vi "Get Track Info.vi"(8 "error in (no error)":errorcluster, 10 "Track Index":i32, 11 "midi file in":refnum<class "midi file.lvclass">) -> (0 "error out":errorcluster, 1 "Track Name":string, 2 "Track Info":T1, 3 "midi file out":refnum<class "midi file.lvclass">)   [LabVIEW 2020, in "midi file.lvclass"]
uses:
  midi file.lvclass
  track info.ctl
  midi file.lvclass/midi file.ctl
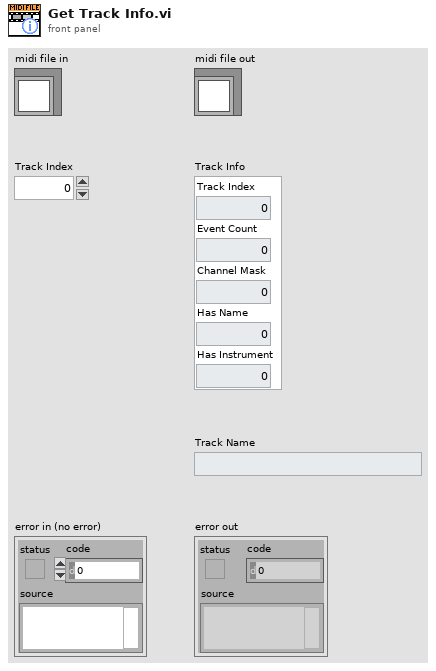
[diagram p1: front panel]
types:
  T1 = typedef "midi file.lvclass/track info.ctl" = cluster{"Track Index":i32, "Event Count":i32, "Channel Mask":i32, "Has Name":i32, "Has Instrument":i32}
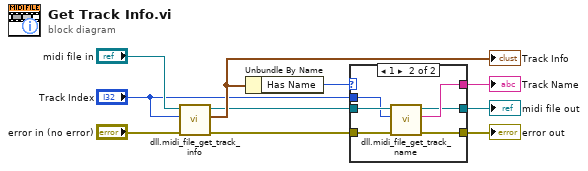
[diagram p0: block diagram]
diagram:
  n1 = call "dll.midi_file_get_track_info.vi"("error in (no error)"="error in (no error)", "Track Index"="Track Index", "midi file in"="midi file in") -> ("error out"=w6:errorcluster, "Track Info"=w8:T1, "midi file out"=w3:refnum<class "midi file.lvclass">)  [unwired: 6 in]
  "Track Info" <- w8
  n2 = Unbundle By Name(w8) -> ("Has Name"=w7:i32)
  n3 = case shown="1" w7 {
    tunnel: w3 -> [w12 w18]
    tunnel: w6 -> [w11 w17]
    tunnel: "Track Index" -> [_ w16]
    tunnel: [_ w15] -> w4
    tunnel: [w12 w14] -> w2
    tunnel: [w11 w13] -> w1
    frame 0, Default {
    }
    frame 1 {
      n4 = call "dll.midi_file_get_track_name.vi"("error in (no error)"=w17, "Track Index"=w16, "midi file in"=w18) -> ("error out"=w13:errorcluster, "Track Name"=w15:string, "midi file out"=w14:refnum<class "midi file.lvclass">)  [unwired: 6 in]
    }
  }
  "error out" <- w1
  "midi file out" <- w2
  "Track Name" <- w4
